vi "MD5Change.vi"(1 "MD5_32":string) -> (0 "MD5_16":string)   [LabVIEW 2013]
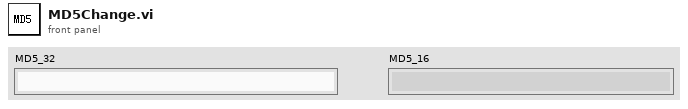
[diagram p1: front panel]
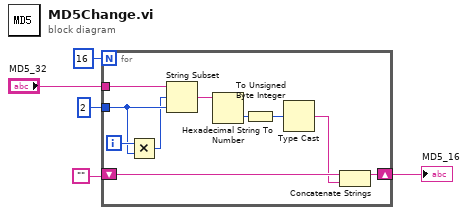
[diagram p0: block diagram]
diagram:
  n1 = for {
    N: 16 -> [_]
    tunnel: "MD5_32" -> [w15]
    tunnel: 2 -> [w13]
    shift-right: [w8] -> w1
    shift-left: "" -> [w7]
    i -> [w14]
    n2 = Multiply(x=w14, y=w13) -> (x*y=w12:i32)
    n3 = String Subset(string=w15, offset (0)=w12, length (rest)=w13) -> (substring=w11:string)
    n4 = Hexadecimal String To Number(string=w11) -> (number=w9:u32)  [unwired: 2 in, 1 out]
    n5 = To Unsigned Byte Integer(number=w9) -> (unsigned 8bit integer=w10:u8)
    n6 = Type Cast(x=w10) -> (*(type *) &x=w6:string)  [unwired: 1 in]
    n7 = Concatenate Strings(w7, w6) -> (w8:string)
  }
  "MD5_16" <- w1
